vi "run_repeating_set_v02.vi"(8 "error in":errorcluster, 9 "data in":T1={"daq_ao 1"="Dev1/ao0", "daq_ai 1"="Dev1/ai0", "experiment day folder"=path "D:/DATA/8-27-15 save func testing/test.lvm", "Multiclamp init error"=0, "Multiclamp Handle Out"=0, "sampling rate (Hz)"=10000, "trial name"=""}, 11 "controls array in":refnum<vi>[](array[refnum])) -> (0 "error out":errorcluster, 1 "data out":T1={"daq_ao 1"="Dev1/ao0", "daq_ai 1"="Dev1/ai0", "experiment day folder"=path "D:/DATA/8-27-15 save func testing/test.lvm", "Multiclamp init error"=0, "Multiclamp Handle Out"=0, "sampling rate (Hz)"=10000, "trial name"=""}, 3 "control array out":refnum<vi>[](array[refnum]))   [LabVIEW 2015]
uses:
  get_data_from_control_tfarray.vi
  get_data_from_control_double.vi
  get_data_from_control_int.vi
  Controls/Data.ctl
panel:
  out "cell quality bad":bool
  out "repeating TF set":T2
  # "RUN REPEATING SET AUTO WC"
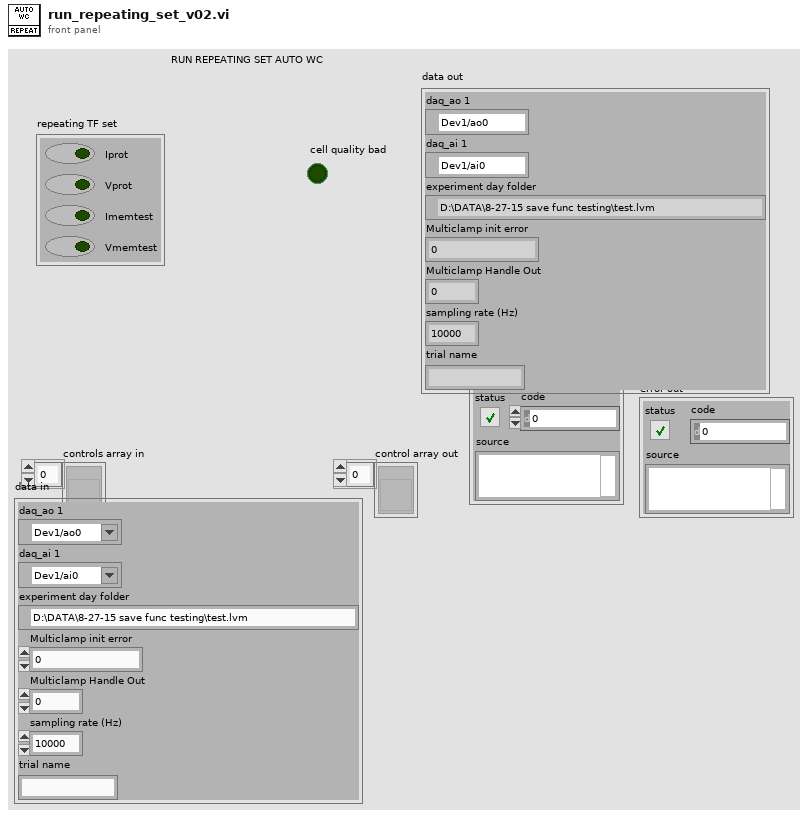
[diagram p1: front panel]
types:
  T1 = typedef "Data.ctl" = cluster{"daq_ao 1":tag, "daq_ai 1":tag, "experiment day folder":path, "Multiclamp init error":i32, "Multiclamp Handle Out":u32, "sampling rate (Hz)":i32, "trial name":string}
  T2 = cluster{" Iprot":bool, " Vprot":bool, " Imemtest":bool, " Vmemtest":bool}
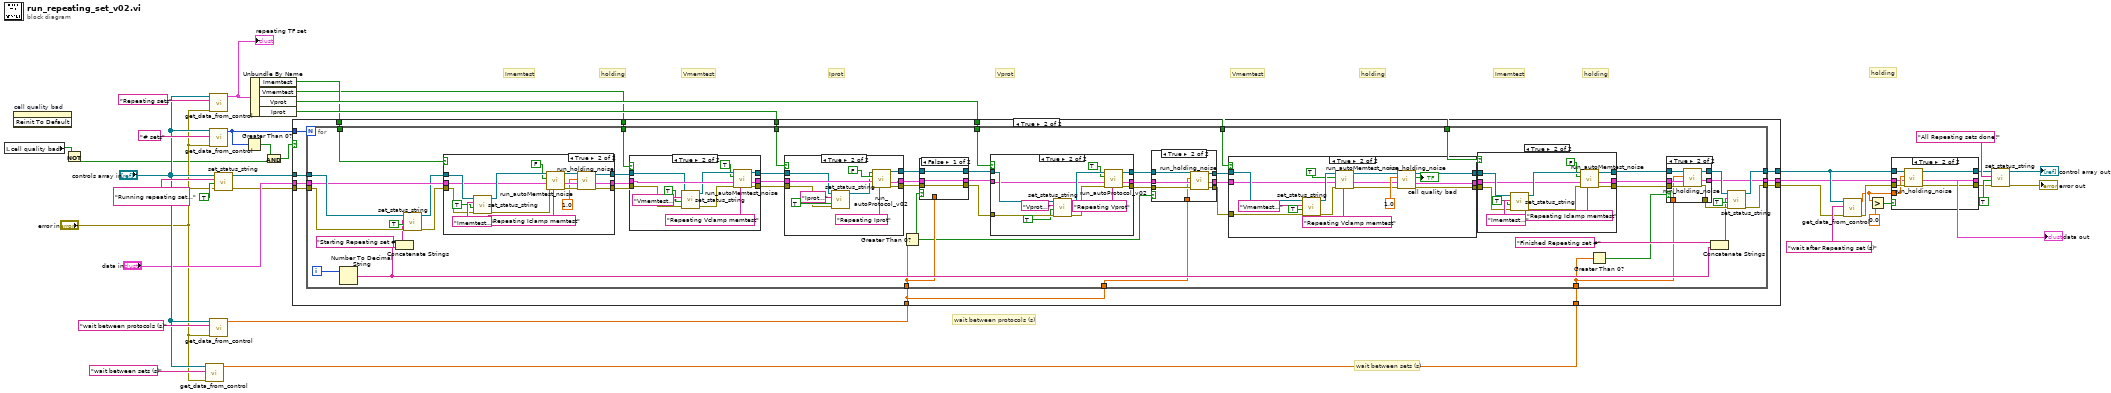
[diagram p0: block diagram]
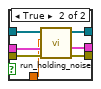
[diagram p5: hidden frame]
diagram:
  # "holding"
  # "wait between sets (s)"
  # "wait between protocols (s)"
  # "Imemtest"
  # "Vmemtest"
  # "holding"
  # "Vmemtest"
  # "holding"
  # "holding"
  # "Imemtest"
  # "Vprot"
  # "Iprot"
  n1 = local read "cell quality bad"() -> (w3:bool)
  n2 = invoke on="cell quality bad" class="Bool (strict)" method="Reinit To Default"() -> ()  [unwired: 3 in, 3 out]
  n3 = Not(x=w3) -> (.not. x?=w4:bool)
  n4 = call-poly "get_data_from_control.vi"("error in"="error in", "control label"="wait between sets (s)", "controls array"="controls array in") -> ("double out"=w15:dbl)  [unwired: 7 in, 1 out]
  n5 = call-poly "get_data_from_control.vi"("error in"="error in", "control label"="Repeating sets", "controls array"="controls array in") -> ("TF set out"=w38:T2)  [unwired: 7 in, 1 out]
  "repeating TF set" <- w38
  n6 = call-poly "get_data_from_control.vi"("error in"="error in", "control label"="# sets", "controls array"="controls array in") -> ("long out"=w12:i32)  [unwired: 7 in, 1 out]
  n7 = call-poly "get_data_from_control.vi"("error in"="error in", "control label"="wait between protocols (s)", "controls array"="controls array in") -> ("double out"=w16:dbl)  [unwired: 7 in, 1 out]
  n8 = call "set_status_string.vi"("error in"="error in", "new line?"=TRUE, "status string in"="Running repeating set...", "controls array"="controls array in") -> ("error out"=w9:errorcluster, "controls array out"=w11:refnum<vi>[])  [unwired: 6 in]
  n9 = Greater Than 0?(x=w12) -> (x > 0?=w2:bool)
  n10 = Unbundle By Name(w38) -> ("Imemtest"=w14:bool, "Vmemtest"=w13:bool, "Vprot"=w30:bool, "Iprot"=w37:bool)
  n11 = And(x=w2, y=w4) -> (x .and. y?=w1:bool)
  n12 = case shown="True" w1 {
    tunnel: w37 -> [_ w54]
    tunnel: w30 -> [_ w53]
    tunnel: w9 -> [w39 w52]
    tunnel: w11 -> [w41 w51]
    tunnel: "data in" -> [w40 w50]
    tunnel: [w41 w49] -> w22
    tunnel: [w39 w48] -> w21
    tunnel: [w40 w47] -> w20
    tunnel: w16 -> [_ w46]
    tunnel: w15 -> [_ w45]
    tunnel: w14 -> [_ w44]
    tunnel: w13 -> [_ w43]
    tunnel: w12 -> [_ w42]
    frame False {
    }
    frame True {
      n13 = for {
        N: w42 -> [_]
        tunnel: w54 -> [w107]
        tunnel: w53 -> [w103]
        tunnel: w44 -> [w68]
        tunnel: w51 -> [w86]
        tunnel: w43 -> [w102]
        tunnel: [w76] -> w49
        tunnel: w52 -> [w83]
        tunnel: [w73] -> w48
        tunnel: w50 -> [w85]
        tunnel: [w74] -> w47
        tunnel: w46 -> [w58]
        tunnel: w46 -> [w59]
        tunnel: w45 -> [w56]
        tunnel: w44 -> [w67]
        tunnel: w43 -> [w66]
        i -> [w79]
        n14 = Number To Decimal String(number=w79) -> (decimal integer string=w70:string)  [unwired: 1 in]
        n15 = Concatenate Strings("Starting Repeating set #" ("status string in"), w70) -> (w78:string)
        n16 = call "set_status_string.vi"("error in"=w83, "new line?"=TRUE, "status string in"=w78, "controls array"=w86) -> ("error out"=w82:errorcluster, "controls array out"=w84:refnum<vi>[])  [unwired: 6 in]
        n17 = case shown="True" w68 {
          tunnel: [w219 w222] -> w63
          tunnel: [w217 w220] -> w65
          tunnel: [w218 w221] -> w64
          tunnel: w82 -> [w217 w229]
          tunnel: w84 -> [w219 w228]
          tunnel: w85 -> [w218 w227]
          frame False {
          }
          frame True {
            n18 = call "set_status_string.vi"("error in"=w229, "new line?"=TRUE, "status string in"="Imemtest...", "controls array"=w228) -> ("error out"=w231:errorcluster, "controls array out"=w234:refnum<vi>[])  [unwired: 6 in]
            n19 = call "run_autoMemtest_noise.vi"("control label"="Repeating Iclamp memtest", "error in"=w231, "data in"=w227, "clamp switch (T=v, F=i)"=FALSE, "controls array"=w234) -> ("error out"=w225:errorcluster, "data out"=w224:T1, "controls out"=w226:refnum<vi>[])  [unwired: 2 in, 2 out]
            n20 = call "run_holding_noise.vi"("error in"=w225, "data in"=w224, "holding time (s)"=1.0, "controls array in"=w226) -> ("error out"=w220:errorcluster, "data out"=w221:T1, "controls array out"=w222:refnum<vi>[])  [unwired: 4 in, 1 out]
          }
        }
        n21 = case shown="True" w102 {
          tunnel: w63 -> [w204 w215]
          tunnel: w65 -> [w202 w211]
          tunnel: w64 -> [w203 w216]
          tunnel: [w204 w209] -> w106
          tunnel: [w203 w208] -> w105
          tunnel: [w202 w207] -> w104
          frame False {
          }
          frame True {
            n22 = call "set_status_string.vi"("error in"=w211, "new line?"=TRUE, "status string in"="Vmemtest...", "controls array"=w215) -> ("error out"=w210:errorcluster, "controls array out"=w214:refnum<vi>[])  [unwired: 6 in]
            n23 = call "run_autoMemtest_noise.vi"("control label"="Repeating Vclamp memtest", "error in"=w210, "data in"=w216, "clamp switch (T=v, F=i)"=TRUE, "controls array"=w214) -> ("error out"=w207:errorcluster, "data out"=w208:T1, "controls out"=w209:refnum<vi>[])  [unwired: 2 in, 2 out]
          }
        }
        n24 = case shown="True" w107 {
          tunnel: w106 -> [w190 w195]
          tunnel: w105 -> [w188 w198]
          tunnel: w104 -> [w189 w199]
          tunnel: [w190 w193] -> w101
          tunnel: [w189 w192] -> w100
          tunnel: [w188 w191] -> w99
          frame False {
          }
          frame True {
            n25 = call "set_status_string.vi"("error in"=w199, "new line?"=TRUE, "status string in"="Iprot...", "controls array"=w195) -> ("controls array out"=w194:refnum<vi>[])  [unwired: 6 in, 1 out]
            n26 = call "run_autoProtocol_v02.vi"("control label"="Repeating Iprot", "data in"=w198, "clamp switch (T=v, F=i)"=FALSE, "controls array"=w194) -> ("error out"=w192:errorcluster, "data out"=w191:T1, "controls array out"=w193:refnum<vi>[])  [unwired: 5 in]
          }
        }
        n27 = Greater Than 0?(x=w58) -> (x > 0?=w57:bool)
        n28 = case shown="False" w57 {
          tunnel: w101 -> [w120 w127]
          tunnel: w100 -> [w118 w126]
          tunnel: w99 -> [w119 w125]
          tunnel: [w120 w124] -> w98
          tunnel: [w119 w123] -> w97
          tunnel: [w118 w122] -> w96
          tunnel: w58 -> [_ w121]
          frame False {
          }
          frame True {
            n29 = call "run_holding_noise.vi"("error in"=w126, "data in"=w125, "holding time (s)"=w121, "controls array in"=w127) -> ("error out"=w122:errorcluster, "data out"=w123:T1, "controls array out"=w124:refnum<vi>[])  [unwired: 4 in, 1 out]
          }
        }
        n30 = case shown="True" w103 {
          tunnel: w98 -> [w155 w167]
          tunnel: w96 -> [w153 w166]
          tunnel: w97 -> [w154 w160]
          tunnel: [w155 w158] -> w95
          tunnel: [w154 w157] -> w93
          tunnel: [w153 w156] -> w94
          frame False {
          }
          frame True {
            n31 = call "set_status_string.vi"("error in"=w166, "new line?"=TRUE, "status string in"="Vprot...", "controls array"=w167) -> ("error out"=w163:errorcluster, "controls array out"=w164:refnum<vi>[])  [unwired: 6 in]
            n32 = call "run_autoProtocol_v02.vi"("control label"="Repeating Vprot", "error in"=w163, "data in"=w160, "clamp switch (T=v, F=i)"=TRUE, "controls array"=w164) -> ("error out"=w156:errorcluster, "data out"=w157:T1, "controls array out"=w158:refnum<vi>[])  [unwired: 4 in]
          }
        }
        n33 = case shown="True" w57 {
          tunnel: w95 -> [w130 w137]
          tunnel: w94 -> [w128 w136]
          tunnel: w93 -> [w129 w135]
          tunnel: [w130 w134] -> w92
          tunnel: [w129 w133] -> w91
          tunnel: [w128 w132] -> w90
          tunnel: w59 -> [_ w131]
          frame False {
          }
          frame True {
            n34 = call "run_holding_noise.vi"("error in"=w136, "data in"=w135, "holding time (s)"=w131, "controls array in"=w137) -> ("error out"=w132:errorcluster, "data out"=w133:T1, "controls array out"=w134:refnum<vi>[])  [unwired: 4 in, 1 out]
          }
        }
        n35 = case shown="True" w66 {
          tunnel: w92 -> [w170 w187]
          tunnel: w90 -> [w168 w185]
          tunnel: w91 -> [w169 w182]
          tunnel: [w170 w172] -> w62
          tunnel: [w168 w175] -> w60
          tunnel: [w169 w174] -> w61
          frame False {
          }
          frame True {
            n36 = call "set_status_string.vi"("error in"=w185, "new line?"=TRUE, "status string in"="Vmemtest...", "controls array"=w187) -> ("error out"=w184:errorcluster, "controls array out"=w186:refnum<vi>[])  [unwired: 6 in]
            n37 = call "run_autoMemtest_noise.vi"("control label"="Repeating Vclamp memtest", "error in"=w184, "data in"=w182, "clamp switch (T=v, F=i)"=TRUE, "controls array"=w186) -> ("error out"=w176:errorcluster, "data out"=w173:T1, "controls out"=w177:refnum<vi>[])  [unwired: 2 in, 2 out]
            n38 = call "run_holding_noise.vi"("error in"=w176, "data in"=w173, "holding time (s)"=1.0, "controls array in"=w177) -> ("error out"=w175:errorcluster, "data out"=w174:T1, "cell quality bad"=→"cell quality bad":bool, "controls array out"=w172:refnum<vi>[])  [unwired: 4 in]
          }
        }
        n39 = case shown="True" w67 {
          tunnel: w62 -> [w140 w152]
          tunnel: w60 -> [w139 w144]
          tunnel: [w140 w148] -> w89
          tunnel: [w139 w147] -> w88
          tunnel: [w138 w146] -> w87
          tunnel: w61 -> [w138 w141]
          frame False {
          }
          frame True {
            n40 = call "set_status_string.vi"("error in"=w144, "new line?"=TRUE, "status string in"="Imemtest...", "controls array"=w152) -> ("error out"=w143:errorcluster, "controls array out"=w150:refnum<vi>[])  [unwired: 6 in]
            n41 = call "run_autoMemtest_noise.vi"("control label"="Repeating Iclamp memtest", "error in"=w143, "data in"=w141, "clamp switch (T=v, F=i)"=FALSE, "controls array"=w150) -> ("error out"=w147:errorcluster, "data out"=w146:T1, "controls out"=w148:refnum<vi>[])  [unwired: 2 in, 2 out]
          }
        }
        n42 = Greater Than 0?(x=w56) -> (x > 0?=w55:bool)
        n43 = case shown="True" w55 {
          tunnel: w89 -> [w108 w117]
          tunnel: w88 -> [w110 w116]
          tunnel: w87 -> [w109 w115]
          tunnel: w56 -> [_ w114]
          tunnel: [w108 w113] -> w77
          tunnel: [w110 w112] -> w75
          tunnel: [w109 w111] -> w74
          frame False {
          }
          frame True {
            n44 = call "run_holding_noise.vi"("error in"=w116, "data in"=w115, "holding time (s)"=w114, "controls array in"=w117) -> ("error out"=w112:errorcluster, "data out"=w111:T1, "controls array out"=w113:refnum<vi>[])  [unwired: 4 in, 1 out]
          }
        }
        n45 = Concatenate Strings("Finished Repeating set #" ("status string in"), w70) -> (w69:string)
        n46 = call "set_status_string.vi"("error in"=w75, "new line?"=TRUE, "status string in"=w69, "controls array"=w77) -> ("error out"=w73:errorcluster, "controls array out"=w76:refnum<vi>[])  [unwired: 6 in]
      }
    }
  }
  n47 = call-poly "get_data_from_control.vi"("error in"=w21, "control label"="wait after Repeating set (s)", "controls array"=w22) -> ("error out"=w24:errorcluster, "double out"=w8:dbl)  [unwired: 7 in]
  n48 = Greater?(x=w8, y=0.0) -> (0:w6:bool)
  n49 = case shown="True" w6 {
    tunnel: [w238 w245] -> w29
    tunnel: [w236 w244] -> w28
    tunnel: [w237 w243] -> w27
    tunnel: w24 -> [w236 w242]
    tunnel: w8 -> [_ w241]
    tunnel: w22 -> [w238 w240]
    tunnel: w20 -> [w237 w239]
    frame False {
    }
    frame True {
      n50 = call "run_holding_noise.vi"("error in"=w242, "data in"=w239, "holding time (s)"=w241, "controls array in"=w240) -> ("error out"=w244:errorcluster, "data out"=w243:T1, "controls array out"=w245:refnum<vi>[])  [unwired: 4 in, 1 out]
    }
  }
  "data out" <- w27
  n51 = call "set_status_string.vi"("error in"=w28, "new line?"=TRUE, "status string in"="All Repeating sets done!", "controls array"=w29) -> ("error out"=→"error out":errorcluster, "controls array out"=→"control array out":refnum<vi>[])  [unwired: 6 in]
